vi "chart_vs_graph.vi"() -> ()   [LabVIEW 2021]
panel:
  out "Waveform Graph":dbl[](graph)
  out "Waveform Chart":dbl(graph)
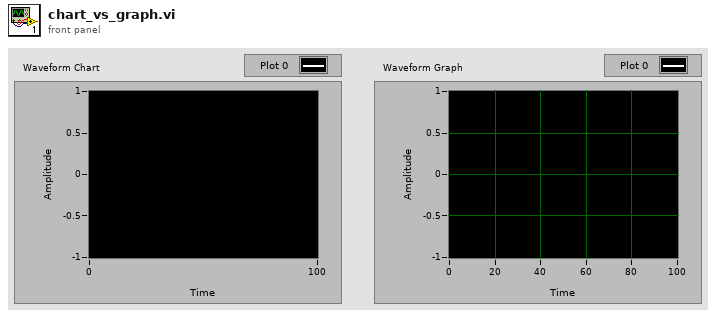
[diagram p1: front panel]
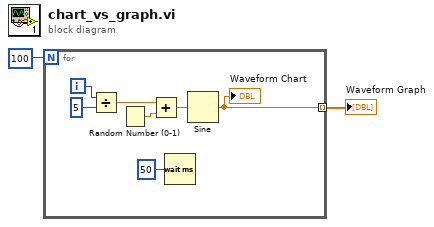
[diagram p0: block diagram]
diagram:
  n1 = for {
    N: 100 -> [_]
    tunnel: [w7] -> w1 mode=indexing
    i -> [w9]
    n2 = Divide(x=w9, y=5) -> (x/y=w5:dbl)
    n3 = Random Number (0-1)() -> (number: 0 to 1=w6:dbl)
    n4 = Add(x=w5, y=w6) -> (x+y=w4:dbl)
    n5 = Wait (ms)(milliseconds to wait=u32 50) -> ()  [unwired: 1 out]
    n6 = Sine(x=w4) -> (sin(x)=w7:dbl)
    "Waveform Chart" <- w7
  }
  "Waveform Graph" <- w1
